vi "GV_timedGraphResizeUpdate.vi"(8 "error in (no error)":errorcluster, 11 "Gviewer in":refnum<class "Gviewer.lvclass">) -> (0 "error out":errorcluster, 3 "Gviewer out":refnum<class "Gviewer.lvclass">)   [LabVIEW 2020, in "Sgraph_lib_V1.lvlib" / "Gviewer.lvclass"]
doc: "Reset the event timer for the graph resize functions"
uses:
  Gviewer.lvclass
  Gviewer.lvclass/Gviewer.ctl
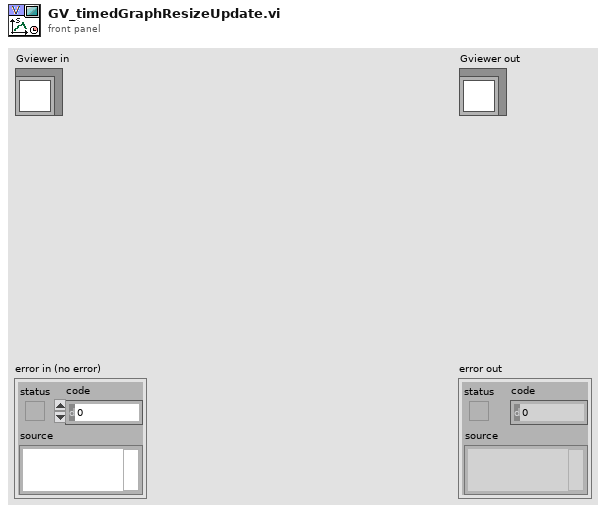
[diagram p1: front panel]
types:
  T1 = typedef "Sgraph_lib_V1.lvlib/Gviewer.lvclass/AttrIdleTimedEvents.ctl" = cluster{"UpdateToolButtons":timestamp, "RedrawGraphUpdate":timestamp, "RequestUpdate":timestamp, "Resize":timestamp}
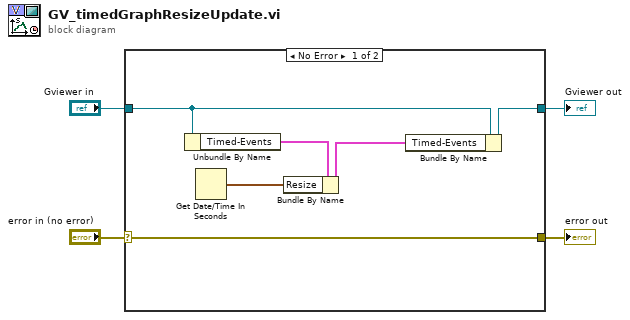
[diagram p0: block diagram]
diagram:
  n1 = case shown="No Error" "error in (no error)" {
    selector: "error in (no error)" -> [w10 w12]
    tunnel: [w10 w12] -> w3
    tunnel: [w6 w11] -> w1
    tunnel: "Gviewer in" -> [w7 w11]
    frame No Error {
      n2 = Unbundle By Name(w7) -> ("Timed-Events"=w9:T1)
      n3 = Get Date/Time In Seconds() -> (seconds since 1Jan1904=w5:timestamp)
      n4 = Bundle By Name(cluster=w9, "Resize"=w5) -> (w8:T1)
      n5 = Bundle By Name(cluster=w7, "Timed-Events"=w8) -> (w6:refnum<class "Gviewer.lvclass">)
    }
    frame Error {
    }
  }
  "error out" <- w3
  "Gviewer out" <- w1
